vi "Init.vi"(8 "Error In":errorcluster, 10 "IConfigure in":refnum<class "IConfigure.lvclass">, 11 "object in":refnum<class "Rigol DS1054.lvclass">) -> (0 "Error Out":errorcluster, 3 "object out":refnum<class "Rigol DS1054.lvclass">)   [LabVIEW 2023]
uses:
  Interfaces/IConfigure/IConfigure.lvclass
  Rigol DS1054.lvclass
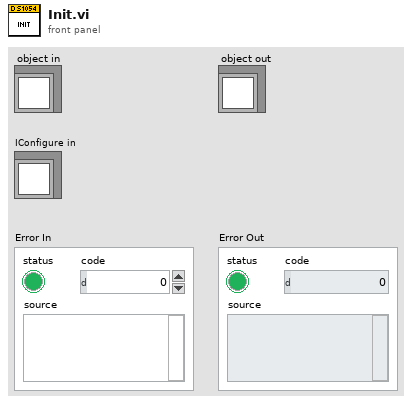
[diagram p1: front panel]
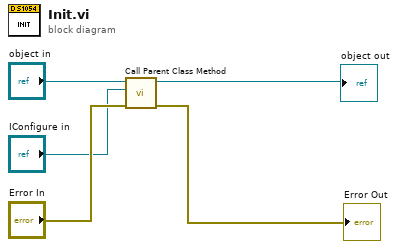
[diagram p0: block diagram]
diagram:
  n1 = call-parent "Call Parent Class Method"("Error In"="Error In", "IConfigure"="IConfigure in", "object in"="object in") -> ("Error Out"=→"Error Out":errorcluster, "object out"=→"object out":refnum<class "Rigol DS1054.lvclass">)  [unwired: 7 in]
